vi "findConer.vi"(0 "Image in":T2, 1 "凹/凸?":bool, 2 "ROI Descriptor":T3={"Global Rectangle"=[1785, 745, 1877, 777], "Contours"=[{"ID"=enum."External", "Type"=12, "Coordinates"=[1785, 745, 1877, 777, 0]}]} {"Contours"."Type" items=["No Selection", "Point", "Line", "Rectangle", "Oval", "Polygon", "Freehand Region", "Annulus", "Unused2", "Unused3", "Broken Line", "Freehand Line", "Rotated Rectangle"]}, 3 "error in":errorcluster, 4 "Search Direction":T1(ring)=enum."Rect Top To Bottom") -> (5 "Image Out":T2(plugin-control), 6 "凹角1":cluster{"X":dbl, "Y":dbl}, 7 "error out":errorcluster)   [LabVIEW 2014]
uses:
  <vilib>/vision/Image Controls.llb/IMAQ Image.ctl
  <vilib>/vision/Contour.llb/IMAQ Connect Range Setting.ctl
  <vilib>/vision/Contour.llb/IMAQ Contour Curve Extraction.ctl
  <vilib>/vision/NI_Vision_Development_Module.lvlib
panel:
  out "Min元素":dbl
  out "Max元素":dbl
  out "波形图表":dbl[](graph)
  in  "File Path":path=path "C:/Users/AICTER/Desktop/Img/4.png"
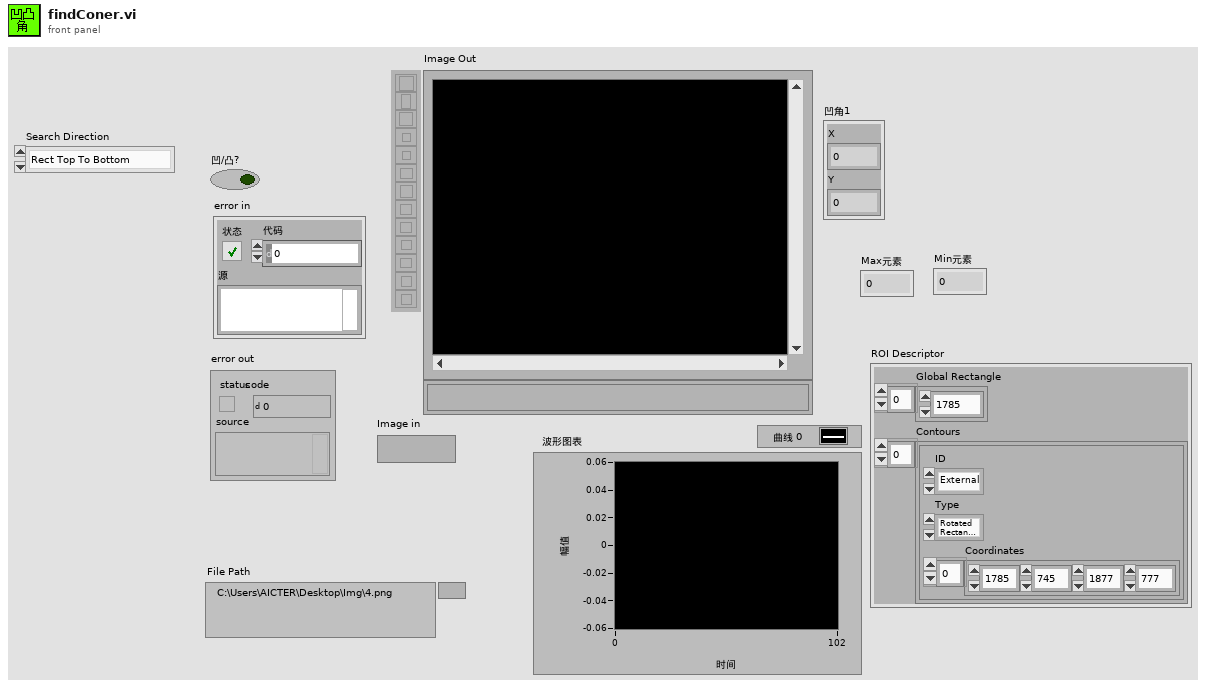
[diagram p1: front panel]
types:
  T1 = enum16{"Rect Left To Right", "Rect Right To Left", "Rect Top To Bottom", "Rect Bottom To Top", "Annulus Inner To Outer", "Annulus Outer To Inner", "Annulus Start Angle To End Angle", "Annulus End Angle To Start Angle"}
  T2 = typedef "IMAQ Image.ctl" = refnum<image>
  T3 = cluster{"Global Rectangle":i32[], "Contours":cluster{"ID":enum32{"External", "Internal"}, "Type":u32, "Coordinates":i32[]}[]}
  T4 = typedef "IMAQ Contour Curve Extraction.ctl" = cluster{"Extraction Mode":u32, "Edge Threshold":i32, "Edge Filter Size":u32, "Min Length":i32, "Search Step Size":i32, "Max Endpoint Gap":i32, "Subpixel":bool}
  T5 = typedef "IMAQ Connect Range Setting.ctl" = cluster{"Match Constraints":u32, "Min":dbl, "Max":dbl}
  T6 = enum16{"Closest To Search Start", "Maximum Length", "Strongest Mean Gradient Change"}
  T7 = cluster{"Overlay?":bool, "Color":u32, "Width":u32, "Maintain Width?":bool}
  T8 = typedef "Image Type" = u32
  T9 = typedef "IMAQ Rectangle" = cluster{"Left":i32, "Top":i32, "Right":i32, "Bottom":i32, "Rotation":dbl}
  T10 = cluster{"Left":i32, "Top":i32, "Right":i32, "Bottom":i32}
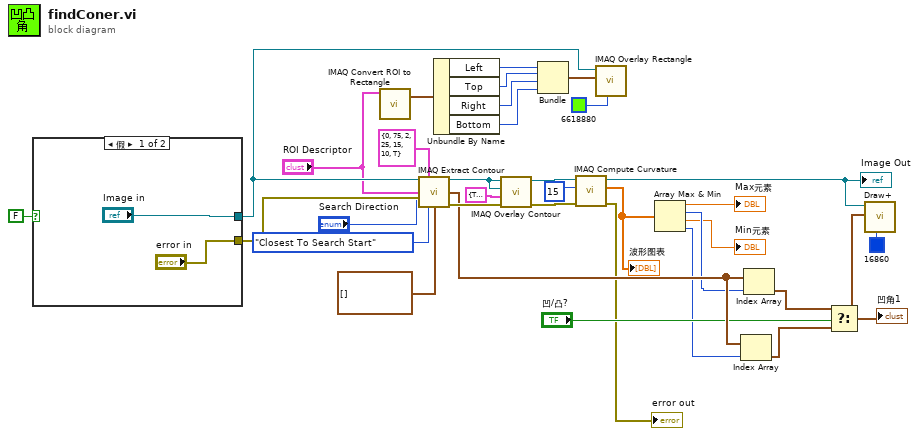
[diagram p0: block diagram]
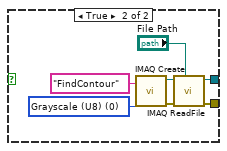
[diagram p2: hidden frame]
diagram:
  n1 = case shown="假" FALSE {
    tunnel: ["error in" w43] -> w34
    tunnel: ["Image in" w39] -> w14
    frame False {
    }
    frame True {
      w40 = T8 0 items=["Grayscale (U8)", "Grayscale (I16)", "Grayscale (SGL)", "Complex (CSG)", "RGB (U32)", "HSL (U32)", "RGB (U64)", "Grayscale (U16)"] ("Image Type")
      n2 = call "IMAQ Create"("Image Name"="FindContour", "Image Type"=w40) -> ("New Image"=w42:T2, "error out"=w41:errorcluster)  [unwired: 2 in, 1 out]
      n3 = call "IMAQ ReadFile"("File Path"="File Path", "error in (no error)"=w41, "Image"=w42) -> ("error out"=w43:errorcluster, "Image Out"=w39:T2)  [unwired: 2 in, 5 out]
    }
  }
  n4 = call "IMAQ Convert ROI to Rectangle"("ROI Descriptor"="ROI Descriptor") -> ("Rectangle"=w20:T9)  [unwired: 8 in, 1 out]
  n5 = call "IMAQ Extract Contour"("Source Image"=w14, "Curve Extraction"=T4 {"Extraction Mode"=0, "Edge Threshold"=75, "Edge Filter Size"=2, "Min Length"=25, "Search Step Size"=15, "Max Endpoint Gap"=10, "Subpixel"=TRUE}, "ROI Descriptor"="ROI Descriptor", "Search Direction"="Search Direction", "error in (no error)"=w34, "Contour Selection"=T6."Closest To Search Start", "Curve Connection"=T5[] []) -> ("Source Image Out"=w27:T2, "Contour Points"=w12:cluster{"X":dbl, "Y":dbl}[], "error out"=w33:errorcluster)  [unwired: 1 in, 5 out]
  n6 = Unbundle By Name(w20) -> ("Left"=w19:i32, "Top"=w18:i32, "Right"=w17:i32, "Bottom"=w16:i32)
  n7 = call "IMAQ Overlay Contour"("error in (no error)"=w33, "Contour Points Settings"=T7 {"Overlay?"=TRUE, "Color"=16711680, "Width"=1, "Maintain Width?"=TRUE}, "Contour Image"=w27, "Image"=w27) -> ("error out"=w31:errorcluster, "Image Out"=w25:T2)  [unwired: 2 in, 4 out]
  n8 = Bundle("Left"=w19, "Top"=w18, "Right"=w17, "Bottom"=w16) -> (w15:T10)  [unwired: 1 in]
  n9 = call "IMAQ Compute Curvature"("error in (no error)"=w31, "Kernel Width"=u32 15, "Contour Image"=w25) -> ("error out"=→"error out":errorcluster, "Curvature Profile (pixel)"=w7:dbl[], "Contour Image Out (dup)"=w23:T2)  [unwired: 1 in, 5 out]
  "Image Out" <- w23
  "波形图表" <- w7
  n10 = call "IMAQ Overlay Rectangle"("Color"=u32 6618880, "Rectangle"=w15, "Image"=w14) -> ()  [unwired: 3 in, 6 out]
  n11 = Array Max & Min(array=w7) -> (max value=→"Max元素":dbl, max index (indices)=w6:i32, min value=→"Min元素":dbl, min index (indices)=w5:i32)
  n12 = Index Array(array=w12, index=w5) -> (element=w10:cluster{"X":dbl, "Y":dbl})
  n13 = Index Array(array=w12, index=w6) -> (element=w11:cluster{"X":dbl, "Y":dbl})
  n14 = Select(t=w11, s="凹/凸?", f=w10) -> (s? t:f=w8:cluster{"X":dbl, "Y":dbl})
  "凹角1" <- w8
  n15 = call "Draw+.vi"("Color"=u32 16860, "input cluster"=w8, "Image In"=w23) -> ()  [unwired: 3 in, 1 out]
